vi "Process.vi"(0 "reference in":refnum<class "Grapher.lvclass">, 5 "error in":errorcluster) -> (14 "reference out":refnum<class "Grapher.lvclass">, 19 "error out":errorcluster)   [LabVIEW 2023, in "Grapher.lvclass"]
uses:
  Grapher.lvclass
  Grapher.lvclass/Grapher.ctl
  <vilib>/Utility/SystemLogging/NI_SystemLogging.lvlib
  <instrlib>/HPS-17000/HPS-17000.lvclass
  <vilib>/HPS-17000/MStream_grpc_CyclerMeasurement.ctl
  <vilib>/HPS-17000/NI_BC_client.lvlib
  Types/Indicators.ctl
panel:
  out "error info":errorcluster
  out "Last Command":string
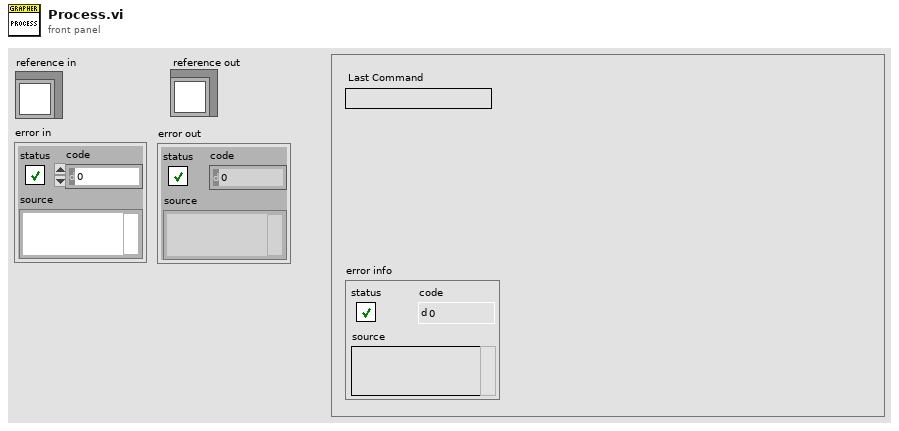
[diagram p1: front panel]
types:
  T1 = typedef "Indicators.ctl" = cluster{"XY Graph":refnum<vi>, "Voltage":refnum<vi>, "Current":refnum<vi>, "Power":refnum<vi>, "Function":refnum<vi>, "Charging":refnum<vi>, "Discharging":refnum<vi>}
  T2 = cluster{"Core":cluster{"Timeout":i32, "Events":cluster{"EventsToProcess":refnum<event-registration>}, "EventFromProcess":refnum<user-event>, "ProcessSyncQueue":refnum<queue>, "QueueFromProcess":refnum<queue>, "Command":string, "Data":variant}, "Chart History":cluster{"local timestamp":dbl[], "system timestamp":dbl[], "measured voltage":dbl[], "measured current":dbl[], "setpoint voltage":dbl[], "setpoint current":dbl[]}, "HPS17K Refs":refnum<class "HPS-17000.lvclass">[], "Use Local Time?":bool, "Graph Samples":u32, "Graph Decimation":i32, "High Speed?":bool, "Graph Queue":refnum<queue>, "Indicator Refs":T1, "Pause?":bool}
  T3 = cluster{"local timestamp":dbl[], "system timestamp":dbl[], "measured voltage":dbl[], "measured current":dbl[], "setpoint voltage":dbl[], "setpoint current":dbl[]}
  T4 = enum32{"Invalid", "Standard", "Closed", "Hidden", "Minimized", "Maximized"}
  T5 = cluster{"EventsToProcess":refnum<event-registration>}
  T6 = typedef "NI_BC_client.lvlib/MStream_grpc_CyclerMeasurement.ctl" = cluster{"measured_voltage":sgl, "measured_current":sgl, "setpoint_voltage":sgl, "setpoint_current":sgl, "timestamp":i64}
  T7 = typedef "Function.ctl" = enum16{"REGEN (LOAD)", "STANDBY", "SUPPLY (SOURCE)"}
  T8 = cluster{"system timestamp":dbl[], "measured voltage":dbl[]}
  T9 = cluster{"system timestamp":dbl[], "setpoint voltage":dbl[]}
  T10 = cluster{"system timestamp":dbl[], "measured current":dbl[]}
  T11 = cluster{"system timestamp":dbl[], "setpoint current":dbl[]}
  T12 = cluster{"system timestamp":dbl[], "setpoint current":dbl[]}[]
  T13 = typedef "Grapher.lvclass/ObjectAttributes.ctl" = cluster{"Indicator Refs":T1, "Update Rate (ms)":i32, "Graph Queue":refnum<queue>, "HPS17K Refs":refnum<class "HPS-17000.lvclass">[]}
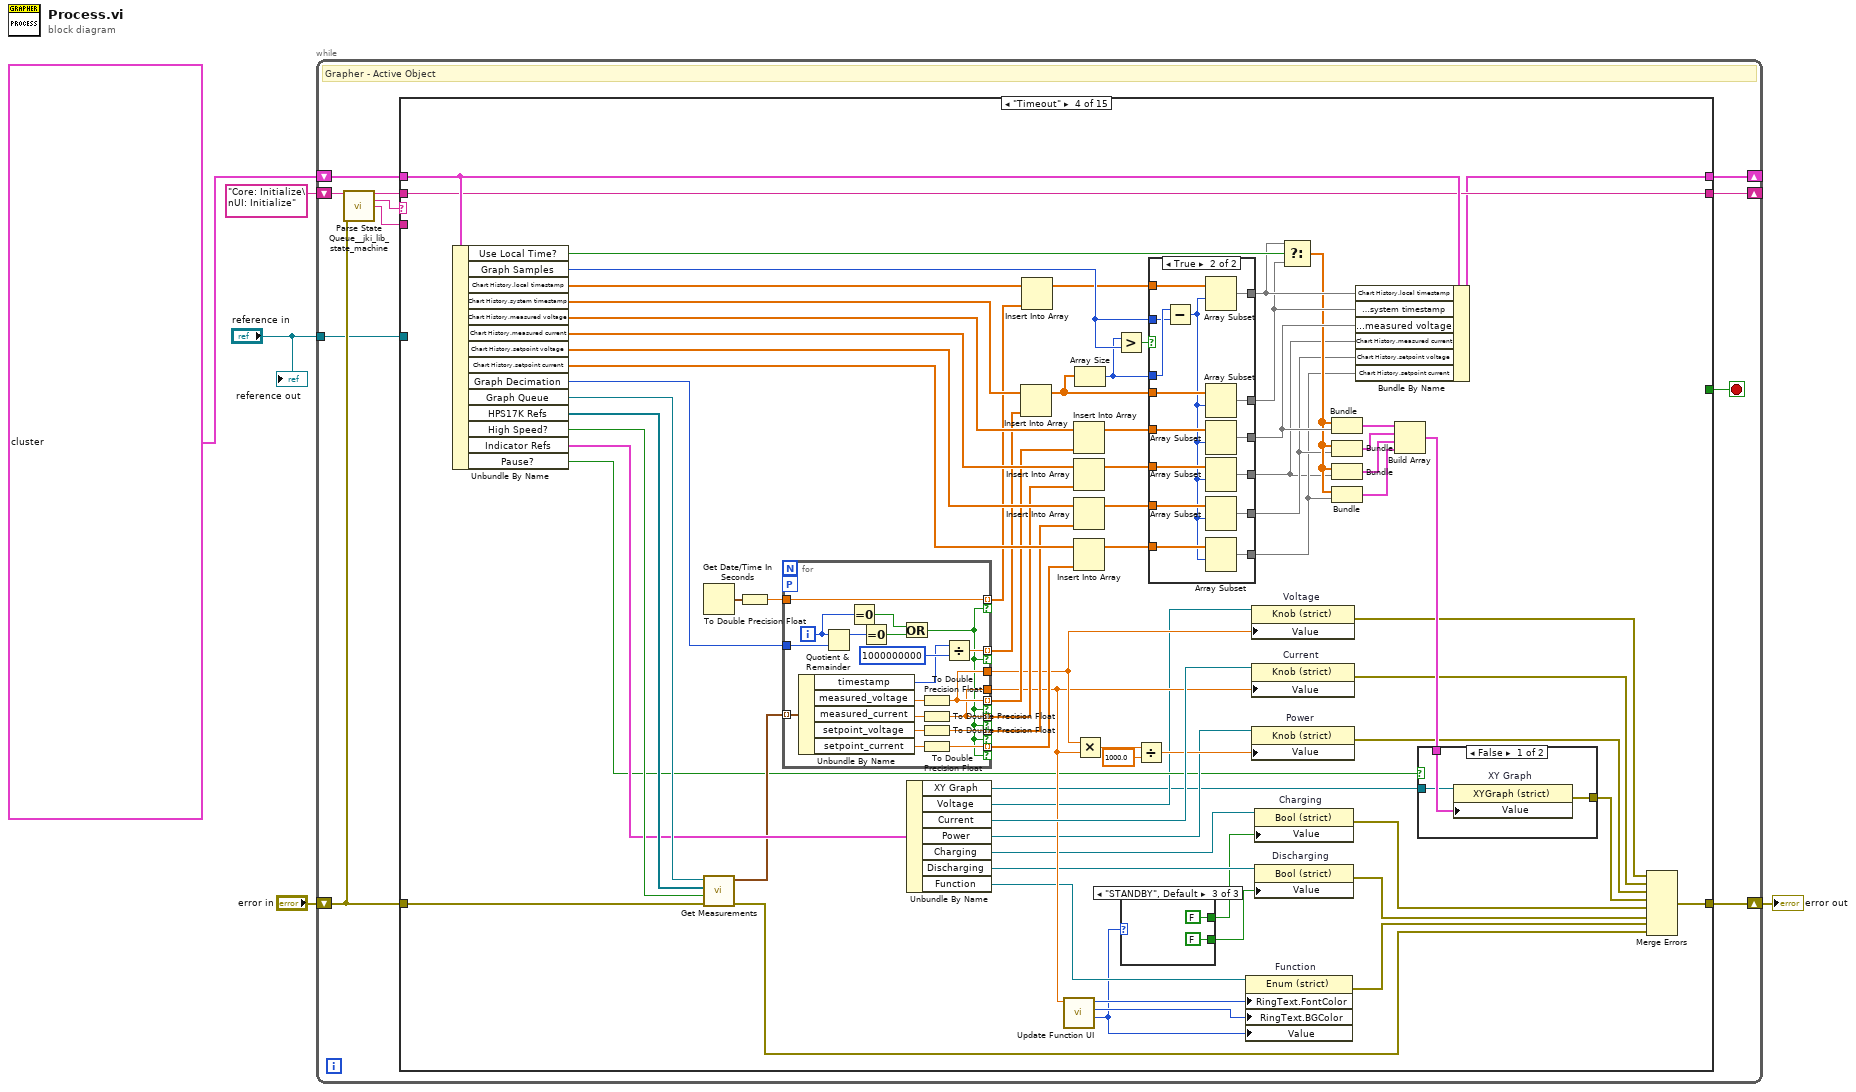
[diagram p0: block diagram]
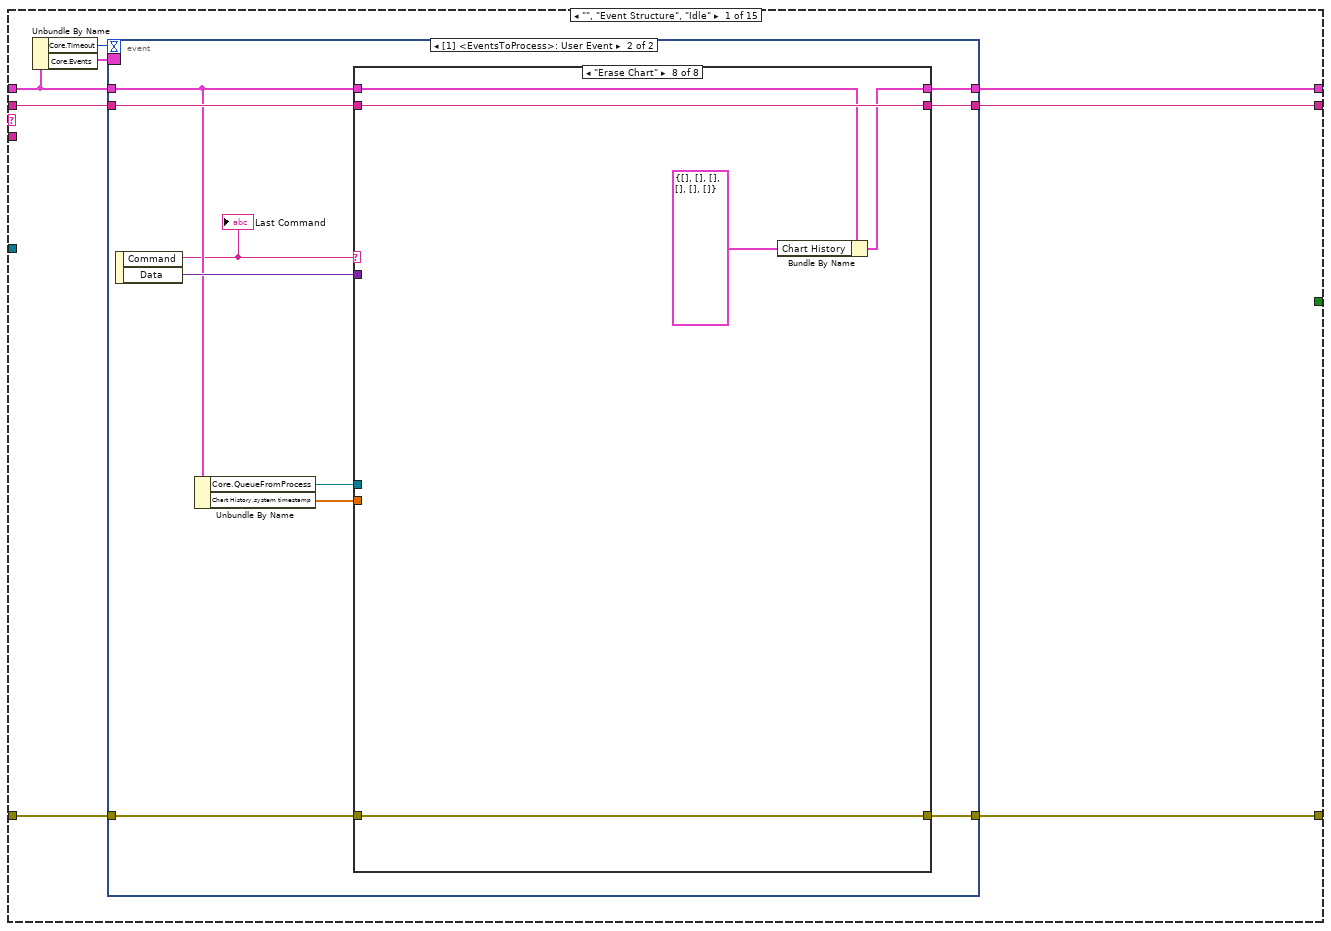
[diagram p2: hidden frame]
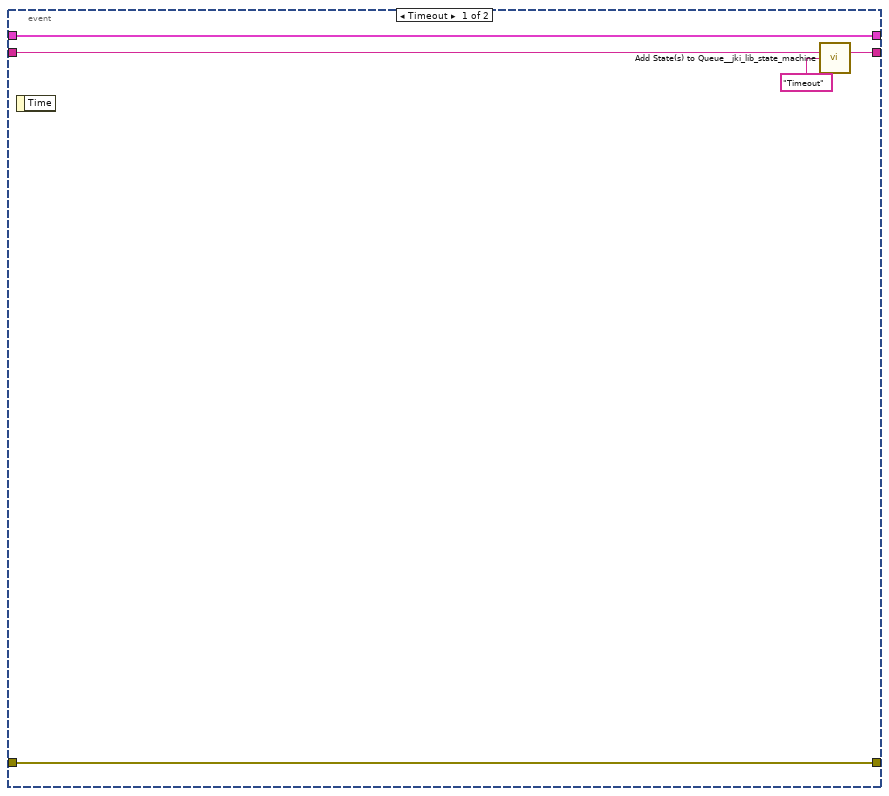
[diagram p3: hidden frame]
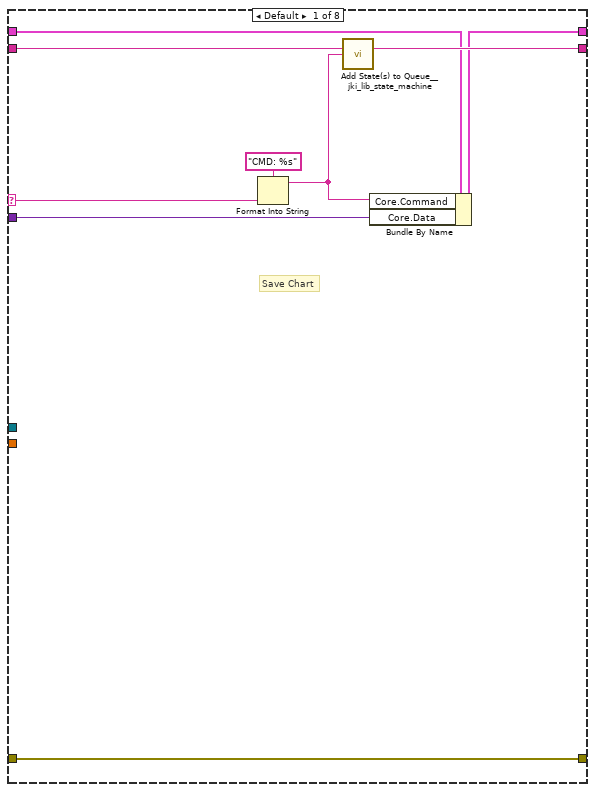
[diagram p4: hidden frame]
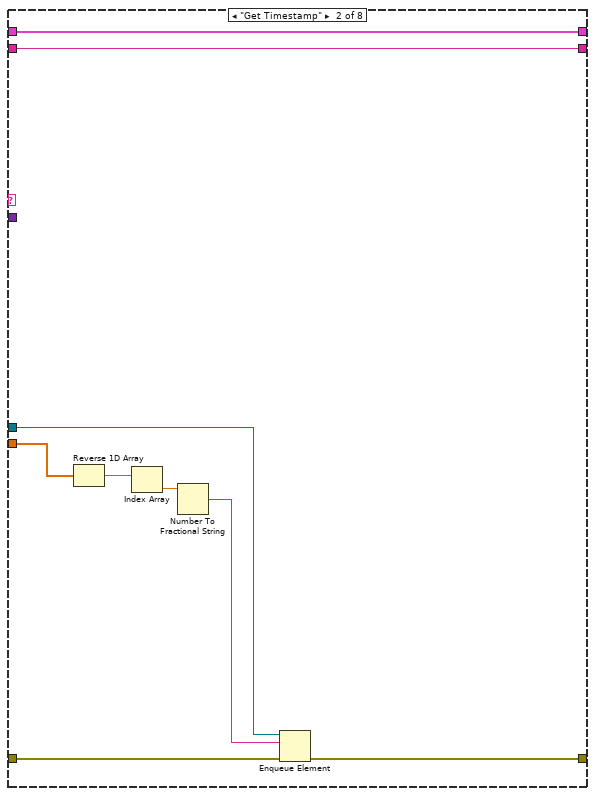
[diagram p5: hidden frame]
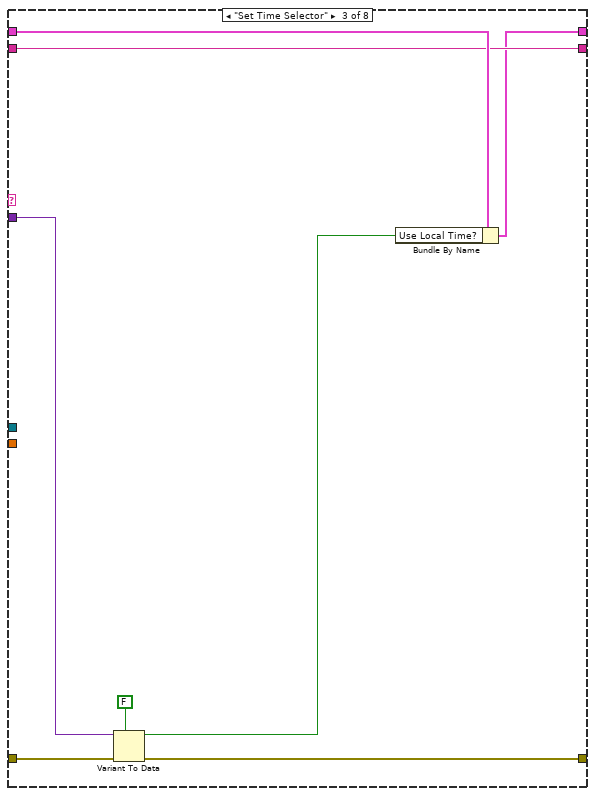
[diagram p6: hidden frame]
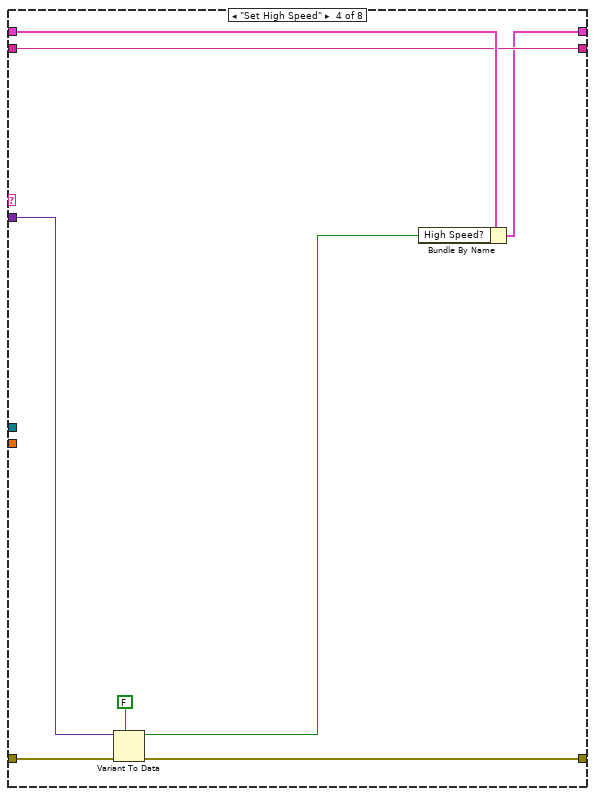
[diagram p7: hidden frame]
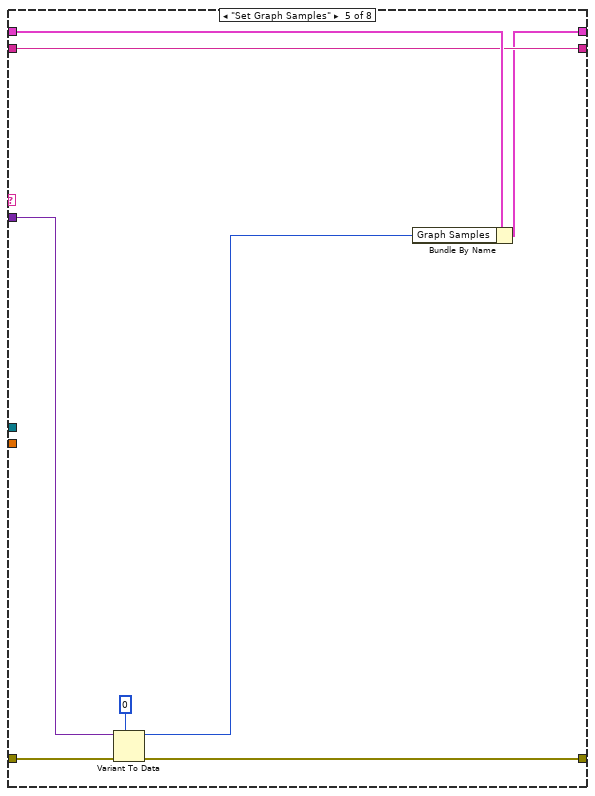
[diagram p8: hidden frame]
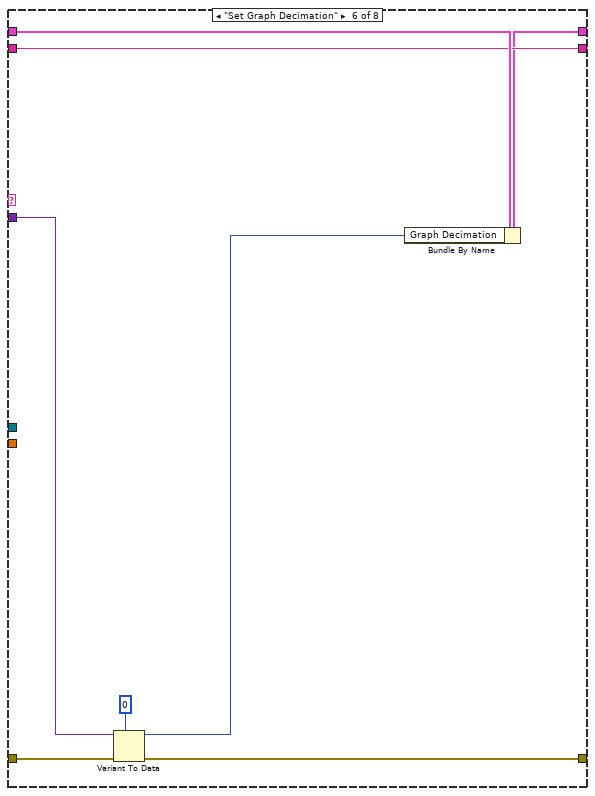
[diagram p9: hidden frame]
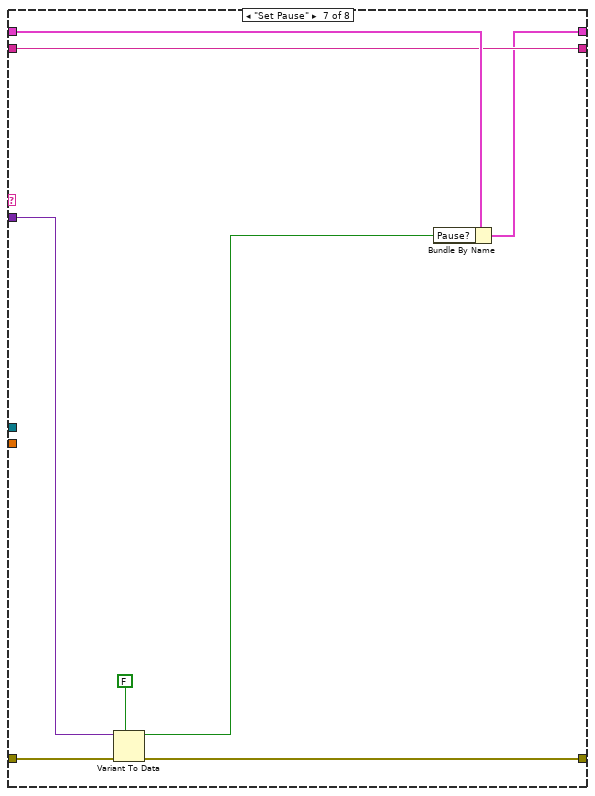
[diagram p10: hidden frame]
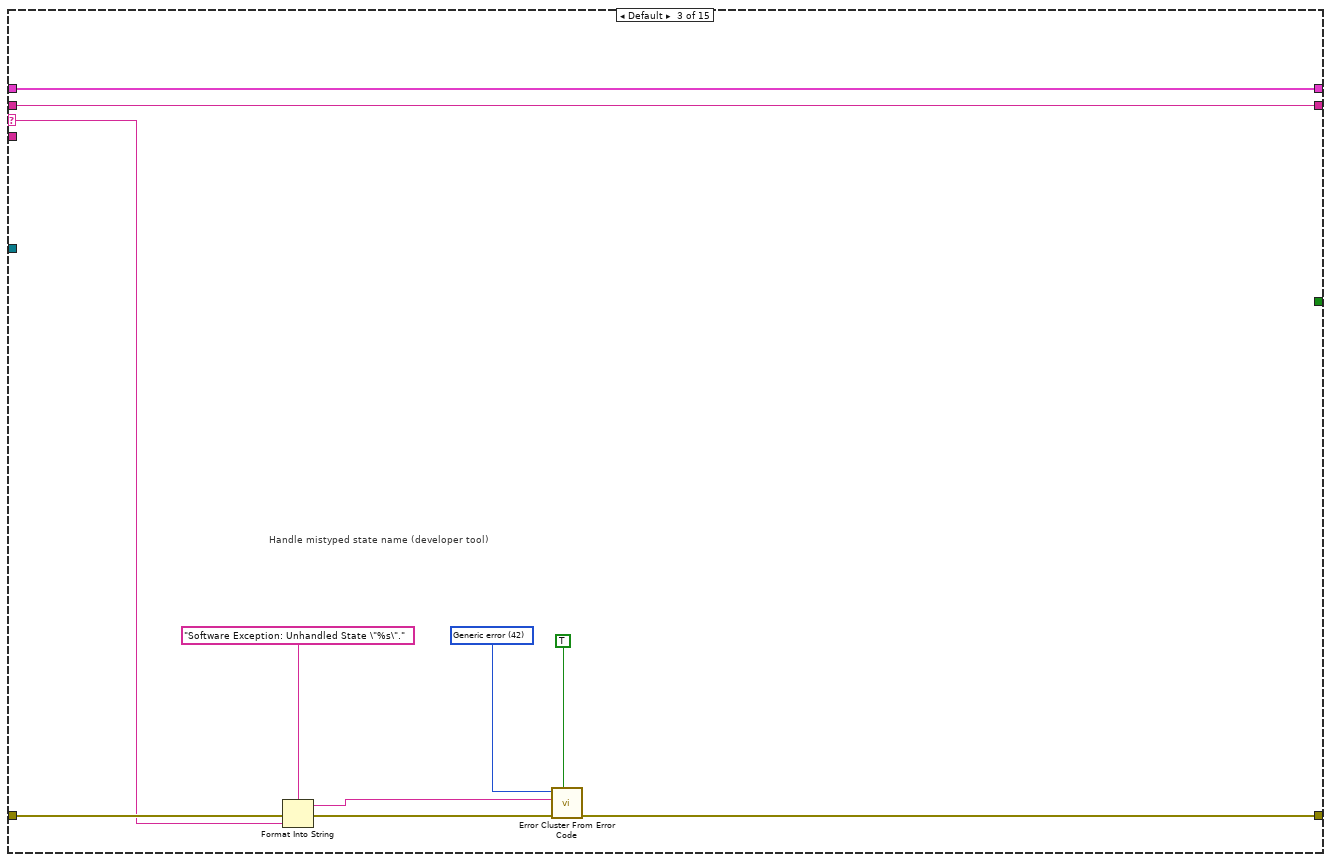
[diagram p12: hidden frame]
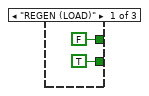
[diagram p13: hidden frame]
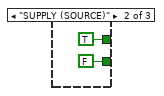
[diagram p14: hidden frame]
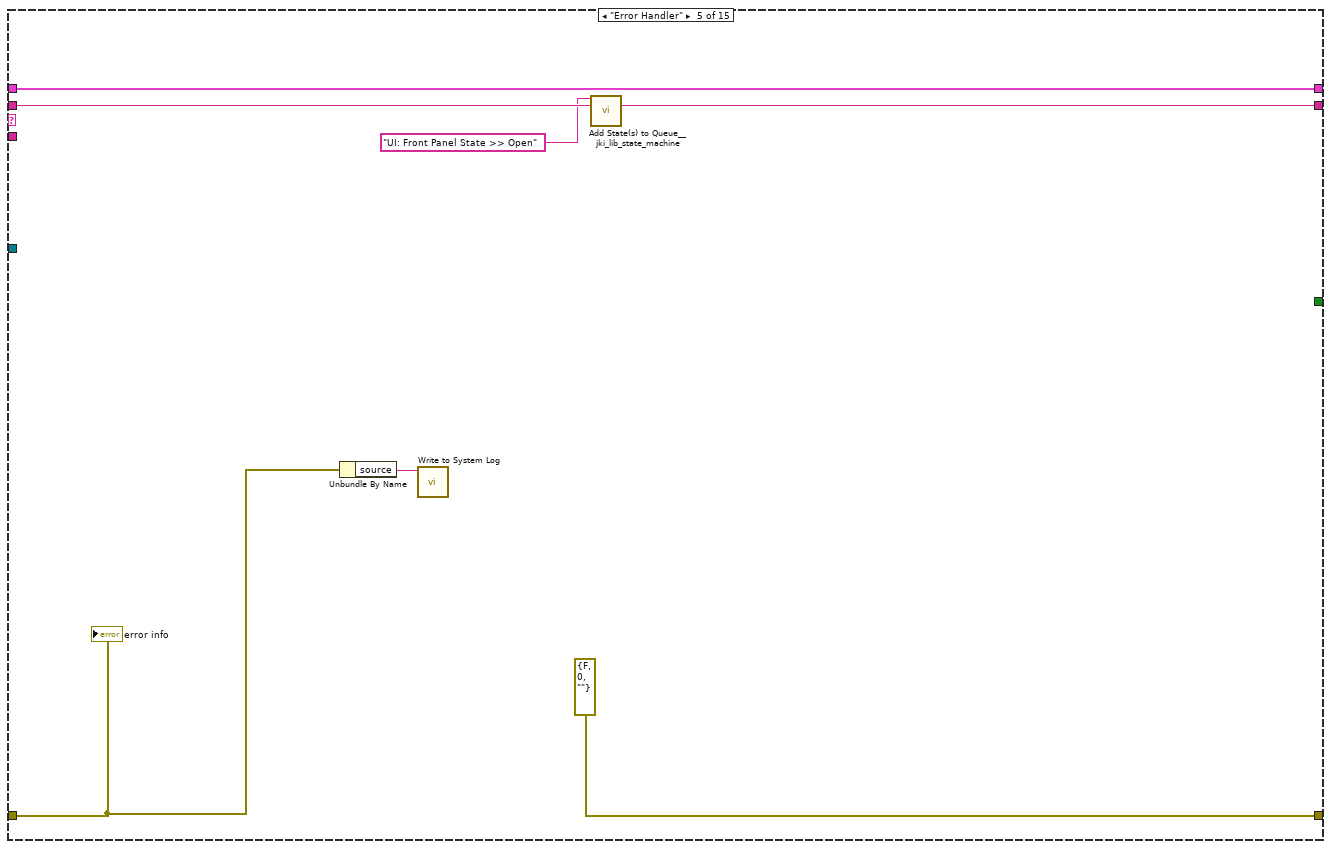
[diagram p17: hidden frame]
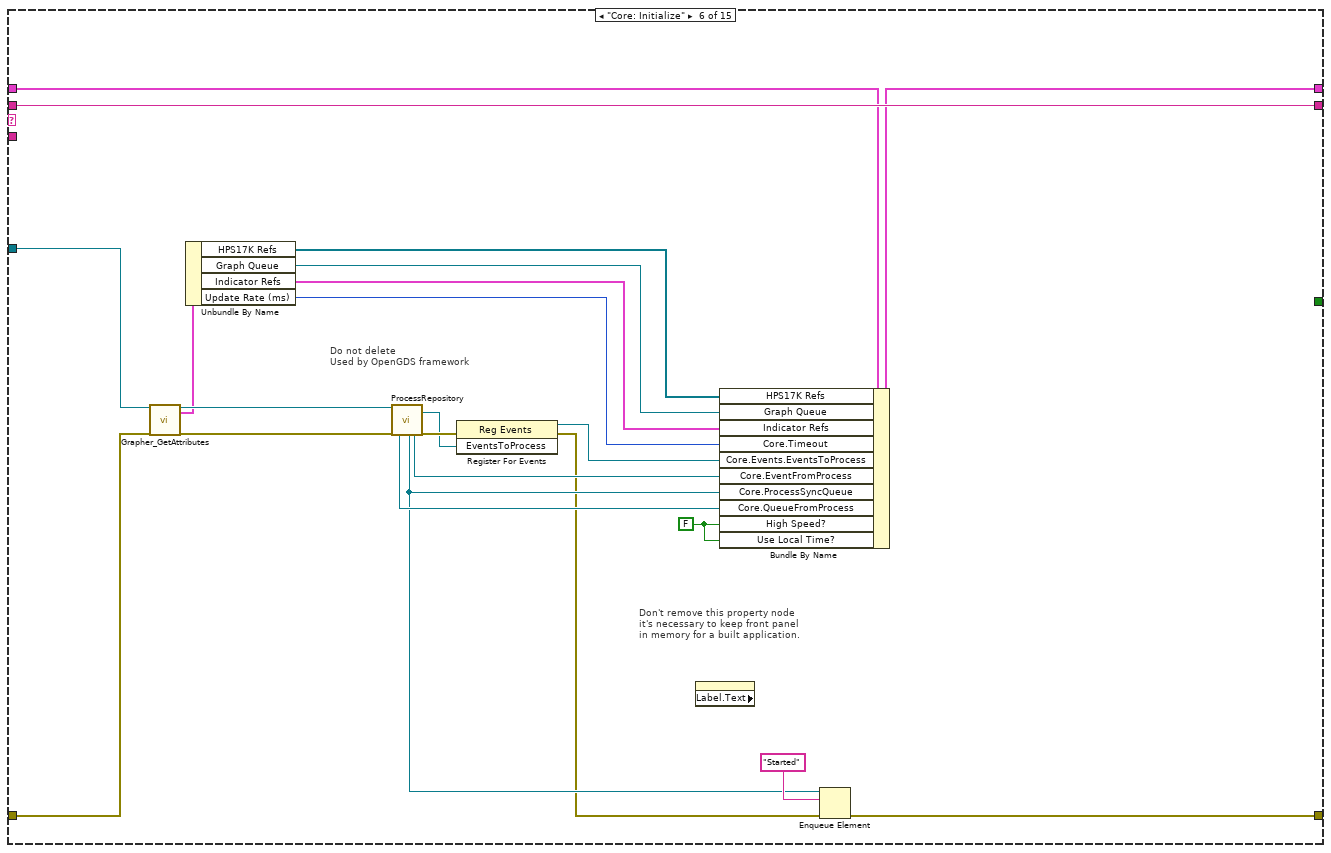
[diagram p18: hidden frame]
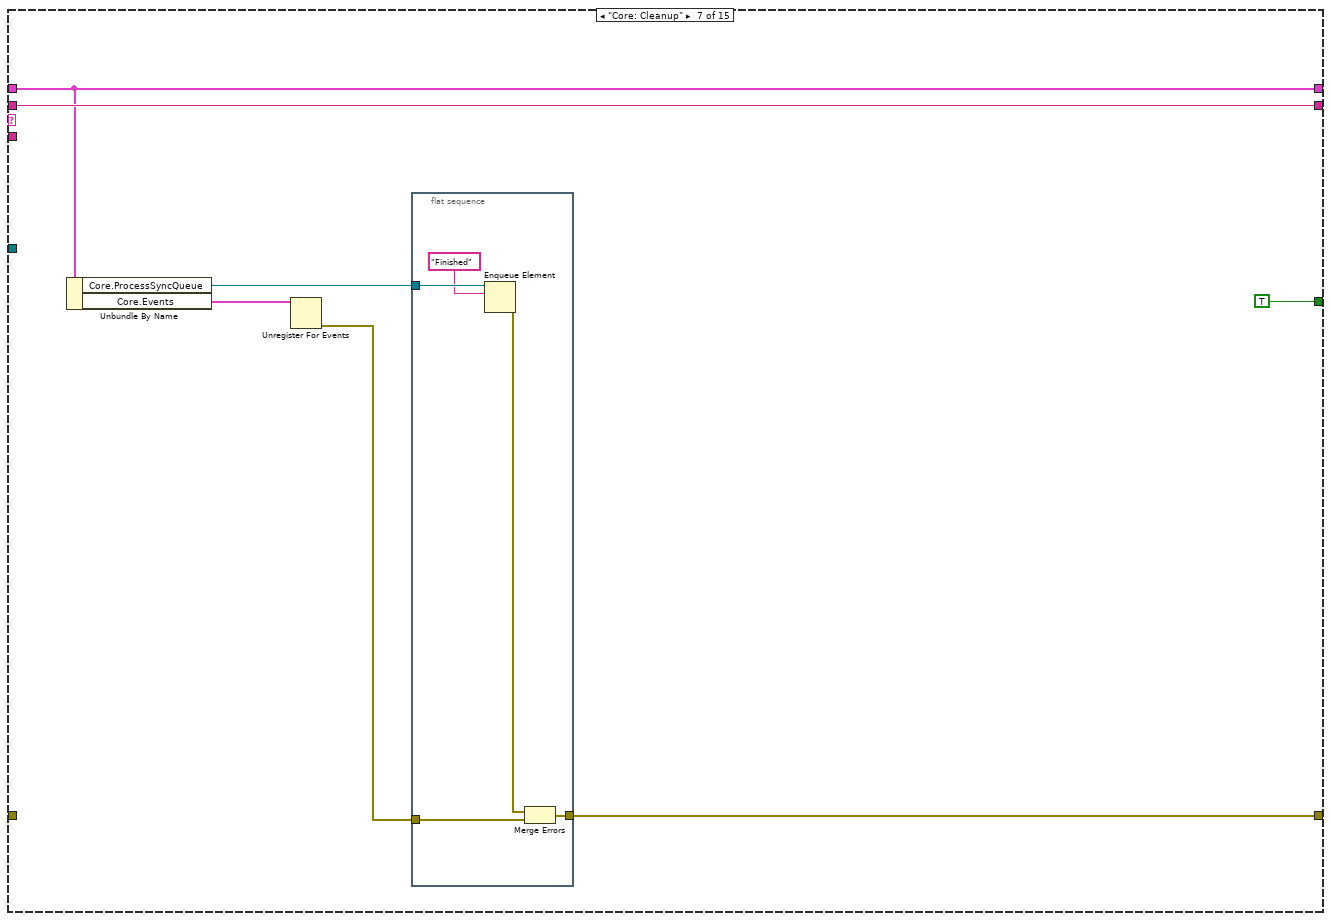
[diagram p19: hidden frame]
diagram:
  n1 = while {
    shift-right: [w15] -> w4
    shift-left: "error in" -> [w16]
    shift-right: [w8] -> _
    shift-left: "Core: Initialize\nUI: Initialize" ("States Out") -> [w11]
    shift-right: [w14] -> _
    shift-left: T2 {"Core"={"Timeout"=-1, "Events"={"EventsToProcess"=refnum}, "EventFromProcess"=refnum, "ProcessSyncQueue"=refnum, "QueueFromProcess"=refnum, "Command"="", "Data"=variant}, "Chart History"={"local timestamp"=[], "system timestamp"=[], "measured voltage"=[], "measured current"=[], "setpoint voltage"=[], "setpoint current"=[]}, "HPS17K Refs"=[], "Use Local Time?"=FALSE, "Graph Samples"=1000, "Graph Decimation"=1000, "High Speed?"=FALSE, "Graph Queue"=refnum, "Indicator Refs"={"XY Graph"=refnum, "Voltage"=refnum, "Current"=refnum, "Power"=refnum, "Function"=refnum, "Charging"=refnum, "Discharging"=refnum}, "Pause?"=FALSE} ("LocalVariables") -> [w13]
    tunnel: "reference in" -> [w6]
    stop <- w7 stop-if-true
    # "Grapher - Active Object"
    n2 = call <vilib>:"Parse State Queue__jki_lib_state_machine.vi"("State Queue"=w11, "Error In (no error)"=w16) -> ("Remaining States"=w10:string, "Current State"=w12:string, "Arguments"=w9:string)  [unwired: 11 in]
    n3 = case shown="\"Timeout\"" w12 {
      selector: w12 -> [_ _ w106 _ _ _ _ _ _ _ _ _ _ _ _]
      tunnel: w16 -> [w18 w105 w108 w187 w240 w254 _ w281 w282 w305 _ w312 w315 w322 w324]
      tunnel: [w19 w105 w107 w186 errorcluster {"status"=FALSE, "code"=0, "source"=""} ("error constant") w266 w269 w281 w282 w305 w306 w312 w315 w322 w323] -> w15
      tunnel: [w24 w104 w115 w184 w244 w264 w270 w280 w284 w297 w307 w311 w314 w321 w326] -> w14
      tunnel: w13 -> [w20 w104 w115 w188 w244 w263 w270 w280 w284 w297 w307 w311 w314 w321 w326]
      tunnel: w10 -> [w22 w103 w114 w185 w243 w265 w273 w279 w285 w304 w309 w310 _ w320 w327]
      tunnel: w9 -> [_ _ _ _ _ _ _ _ w283 _ _ _ _ w317 _]
      tunnel: [w21 w103 w114 w185 w242 w265 w273 w279 w285 w304 w309 w310 "UI: Cleanup\nCore: Cleanup" ("State(s) at Back (\"\")") w319 w327] -> w8
      tunnel: [_ _ _ _ _ _ TRUE _ _ _ _ _ _ _ _] -> w7
      tunnel: w6 -> [_ _ _ _ _ w252 _ _ _ _ _ _ _ _ _]
      frame "", "Event Structure", "Idle" {
        n4 = Unbundle By Name(w20) -> ("Core.Timeout"=w17:i32, "Core.Events"=w23:T5)
        n5 = event shown="[1] <EventsToProcess>: User Event" {
          selector: w23 -> [_ _]
          dyn-events: _ -> [_ _]
          timeout: w17 -> [_ _]
          tunnel: w20 -> [w29 w34]
          tunnel: [w29 w37] -> w24
          tunnel: [w27 w39] -> w21
          tunnel: w22 -> [w28 w38]
          tunnel: [w25 w30] -> w19
          tunnel: w18 -> [w25 w31]
          event Timeout {
            n6 = event-data() -> ()  [unwired: 1 in, 1 out]
            n7 = call <vilib>:"Add State(s) to Queue__jki_lib_state_machine.vi"("State(s) in (\"\")"=w28, "State(s) at Back (\"\")"="Timeout" ("State(s) at Back (\"\")")) -> ("States Out"=w27:string)  [unwired: 13 in]
          }
          event User Event {
            n8 = event-data() -> ("Command"=w33:string, "Data"=w36:variant)  [unwired: 1 in]
            "Last Command" <- w33
            n9 = Unbundle By Name(w34) -> ("Core.QueueFromProcess"=w35:refnum<queue>, "Chart History.system timestamp"=w32:dbl[])
            n10 = case shown="\"Erase Chart\"" w33 {
              selector: w33 -> [w41 _ _ _ _ _ _ _]
              tunnel: [w48 w55 w62 w70 w78 w86 w94 w102] -> w39
              tunnel: w38 -> [w47 w55 w62 w70 w78 w86 w94 w102]
              tunnel: [w46 w56 w59 w67 w77 w85 w93 w100] -> w37
              tunnel: w36 -> [w45 _ w64 w72 w80 w88 w96 _]
              tunnel: w35 -> [_ w57 _ _ _ _ _ _]
              tunnel: w34 -> [w44 w56 w63 w71 w79 w87 w95 w101]
              tunnel: w32 -> [_ w53 _ _ _ _ _ _]
              tunnel: w31 -> [w40 w54 w65 w73 w81 w89 w97 w99]
              tunnel: [w40 w49 w58 w66 w76 w84 w92 w99] -> w30
              frame Default {
                # "Save Chart"
                n11 = Format Into String(format string="CMD: %s", w41) -> (resulting string=w42:string)  [unwired: 2 in, 1 out]
                n12 = call <vilib>:"Add State(s) to Queue__jki_lib_state_machine.vi"("State(s) in (\"\")"=w47, "State(s) at Back (\"\")"=w42) -> ("States Out"=w48:string)  [unwired: 13 in]
                n13 = Bundle By Name(cluster=w44, "Core.Command"=w42, "Core.Data"=w45) -> (w46:T2)
              }
              frame "Get Timestamp" {
                n14 = Reverse 1D Array(array=w53) -> (reversed array=w52:dbl[])
                n15 = Index Array(array=w52) -> (element=w51:dbl)  [unwired: 1 in]
                n16 = Number To Fractional String(number=w51) -> (F-format string=w50:string)  [unwired: 3 in]
                n17 = Enqueue Element ("Return message to the client from this process")(queue=w57, element=w50, error in (no error)=w54) -> (error out=w49:errorcluster)  [unwired: 1 in, 2 out]
              }
              frame "Set Time Selector" {
                n18 = Variant To Data(error in=w65, type=FALSE, Variant=w64) -> (data=w61:bool, error out=w58:errorcluster)
                n19 = Bundle By Name(cluster=w63, "Use Local Time?"=w61) -> (w59:T2)
              }
              frame "Set High Speed" {
                n20 = Variant To Data(error in=w73, type=FALSE, Variant=w72) -> (data=w69:bool, error out=w66:errorcluster)
                n21 = Bundle By Name(cluster=w71, "High Speed?"=w69) -> (w67:T2)
              }
              frame "Set Graph Samples" {
                n22 = Variant To Data(error in=w81, type=u32 0 ("Graph Samples"), Variant=w80) -> (data=w74:u32, error out=w76:errorcluster)
                n23 = Bundle By Name(cluster=w79, "Graph Samples"=w74) -> (w77:T2)
              }
              frame "Set Graph Decimation" {
                n24 = Variant To Data(error in=w89, type=0 ("Graph Samples"), Variant=w88) -> (data=w82:i32, error out=w84:errorcluster)
                n25 = Bundle By Name(cluster=w87, "Graph Decimation"=w82) -> (w85:T2)
              }
              frame "Set Pause" {
                n26 = Variant To Data(error in=w97, type=FALSE, Variant=w96) -> (data=w91:bool, error out=w92:errorcluster)
                n27 = Bundle By Name(cluster=w95, "Pause?"=w91) -> (w93:T2)
              }
              frame "Erase Chart" {
                n28 = Bundle By Name(cluster=w101, "Chart History"=T3 {"local timestamp"=[], "system timestamp"=[], "measured voltage"=[], "measured current"=[], "setpoint voltage"=[], "setpoint current"=[]}) -> (w100:T2)
              }
            }
          }
        }
      }
      frame "---------- Core ----------" {
      }
      frame Default {
        w112 = 42 items=["No error", "Argument error", "Memory is full", "Out of zone", "End of file", "File already open", "Generic file I/O error", "File not found", "File permission error", "Disk is full", "Duplicate path", "Too many files open", "System feature not enabled", "Resource file not found", "Cannot add resource", "Resource not found", "Image not found", "Image memory error", "Pen does not exist", "Config type invalid", "Config token not found", "Config parse error", "Config memory error", "Bad external code format", "Bad external code offset", "External code not present", "Null window", "Destroy window error", "Null menu", "Print aborted", "Bad print record", "Print driver error", "Windows error during printing", "Memory error during printing", "Print dialog error", "Generic print error", "Invalid device refnum", "Device not found", "Device parameter error", "Device unit error", "Cannot open device", "Device call aborted", "Generic error", "Cancelled by user", "Object ID too low", "Object ID too high", "Object not in heap", "Unknown heap", "Unknown object (invalid DefProc)", "Unknown object (DefProc not in table)", "Message out of range", "Invalid (null) method", "Unknown message", "Manager call not supported", "Bad address", "Network operation in progress", "Network operation timed out", "Connection is busy", "Network attribute not supported", "Network error", "Address in use", "System out of memory", "Connection aborted", "Connection refused", "Not connected", "Already connected", "Connection closed", "Initialization error (interapplication manager)", "Bad occurrence", "Wait on unbound occurrence handler", "Occurrence queue overflow", "Datalog type conflict", "Unused", "Unrecognized type (interapplication manager)", "Memory corrupt", "Failed to make temporary DLL", "Old CIN version", "Drag socket not found", "Failed to load drop-object", "Failed to register OLE object", "Failed to release OLE object", "Format specifier type mismatch", "Unknown format specifier", "Too few format specifiers", "Too many format specifiers", "Scan failed", "Newer CIN version", "Error converting to variant", "Runtime menu error", "Password tampered", "Variant attribute not found", "Incompatible variant data type", "Event data is not available", "Event Store is not present", "Occurrence is not found", "Event Queue is not created", "Event info is not available", "Refnum passed is NULL", "Error retrieving Class GUID", "Error retrieving CoClass GUID", "Error retrieving TypeLib GUID.", "Bad built application magic bytes.", "Specific driver is different from the specific driver associated with the Logical Name.", "There is no session opened to the class driver.", "Max Error", "MAX - Error with config objects", "MAX - Error loading configuration", "MAX - Group not supported"]
        # "Handle mistyped state name (developer tool)"
        n29 = Format Into String(format string="Software Exception: Unhandled State \"%s\"." ("message"), error in=w108, w106) -> (resulting string=w111:string, error out=w110:errorcluster)  [unwired: 1 in]
        n30 = call <vilib>:"Error Cluster From Error Code.vi"("show call chain? (False)"=TRUE, "error in (no error)"=w110, "error message (\"\")"=w111, "error code (0)"=w112) -> ("error out"=w107:errorcluster)  [unwired: 5 in]
      }
      frame "Timeout" {
        n31 = Unbundle By Name(w188) -> ("Use Local Time?"=w171:bool, "Graph Samples"=w183:u32, "Chart History.local timestamp"=w182:dbl[], "Chart History.system timestamp"=w181:dbl[], "Chart History.measured voltage"=w180:dbl[], "Chart History.measured current"=w179:dbl[], "Chart History.setpoint voltage"=w178:dbl[], "Chart History.setpoint current"=w177:dbl[], "Graph Decimation"=w176:i32, "Graph Queue"=w175:refnum<queue>, "HPS17K Refs"=w174:refnum<class "HPS-17000.lvclass">[], "High Speed?"=w173:bool, "Indicator Refs"=w172:T1, "Pause?"=w128:bool)
        n32 = Get Date/Time In Seconds() -> (seconds since 1Jan1904=w163:timestamp)
        n33 = call "Get Measurements.vi"("error in (no error)"=w187, "High Speed"=w173, "HPS17K Refs"=w174, "Stream Queue"=w175) -> ("error out"=w122:errorcluster, "Measurements"=w148:T6[])  [unwired: 6 in]
        n34 = To Double Precision Float(number=w163) -> (double precision float=w142:dbl)
        n35 = for {
          tunnel: w148 -> [w216] mode=indexing
          tunnel: [w206] -> w143 mode=indexing if=w198
          tunnel: [w205] -> w144 mode=indexing if=w198
          tunnel: [w210] -> w154 mode=indexing if=w198
          tunnel: [w209] -> w153 mode=indexing if=w198
          tunnel: [w207] -> w149 mode=indexing if=w198
          workers-P: _ -> [_]
          tunnel: [w206] -> w137
          tunnel: [w205] -> w135
          tunnel: w176 -> [w204]
          tunnel: w142 -> [w199]
          tunnel: [w199] -> w141 mode=indexing if=w198
          i -> [w201]
          n36 = Unbundle By Name(w216) -> ("timestamp"=w208:i64, "measured_voltage"=w214:sgl, "measured_current"=w213:sgl, "setpoint_voltage"=w212:sgl, "setpoint_current"=w211:sgl)
          n37 = Quotient & Remainder(x=w201, y=w204) -> (x-y*floor(x/y)=w203:i32)  [unwired: 1 out]
          n38 = Equal To 0?(x=w201) -> (x = 0?=w200:bool)
          n39 = Equal To 0?(x=w203) -> (x = 0?=w202:bool)
          n40 = Or(x=w200, y=w202) -> (x .or. y?=w198:bool)
          n41 = To Double Precision Float(number=w214) -> (double precision float=w206:dbl)
          n42 = To Double Precision Float(number=w213) -> (double precision float=w205:dbl)
          n43 = To Double Precision Float(number=w212) -> (double precision float=w207:dbl)
          n44 = To Double Precision Float(number=w211) -> (double precision float=w210:dbl)
          n45 = Divide(x=w208, y=i64 1000000000) -> (x/y=w209:dbl)
        }
        n46 = Unbundle By Name(w172) -> ("XY Graph"=w124:refnum<vi>, "Voltage"=w125:refnum<vi>, "Current"=w136:refnum<vi>, "Power"=w133:refnum<vi>, "Charging"=w123:refnum<vi>, "Discharging"=w126:refnum<vi>, "Function"=w127:refnum<vi>)
        n47 = Insert Into Array(array=w181, new element=w153) -> (w151:dbl[])  [unwired: 1 in]
        n48 = Insert Into Array(array=w182, new element=w141) -> (w152:dbl[])  [unwired: 1 in]
        n49 = call "Update Function UI.vi"("measured_current"=w135) -> ("Function"=w118:T7, "BG Color"=w139:u32, "Font Color"=w140:u32)  [unwired: 8 in]
        n50 = Insert Into Array(array=w180, new element=w143) -> (w158:dbl[])  [unwired: 1 in]
        n51 = Insert Into Array(array=w179, new element=w144) -> (w157:dbl[])  [unwired: 1 in]
        n52 = Insert Into Array(array=w178, new element=w149) -> (w156:dbl[])  [unwired: 1 in]
        n53 = Insert Into Array(array=w177, new element=w154) -> (w155:dbl[])  [unwired: 1 in]
        n54 = Array Size(array=w151) -> (size(s)=w150:i32)
        n55 = Multiply(x=w137, y=w135) -> (x*y=w170:dbl)
        n56 = Greater?(x=w150, y=w183) -> (0:w159:bool)
        n57 = case shown="\"STANDBY\", Default" w118 {
          tunnel: [TRUE FALSE FALSE] -> w117
          tunnel: [FALSE TRUE FALSE] -> w116
          frame "REGEN (LOAD)" {
          }
          frame "SUPPLY (SOURCE)" {
          }
          frame "STANDBY", Default {
          }
        }
        n58 = Divide(x=w170, y=1000.0) -> (x/y=w134:dbl)
        n59 = case shown="True" w159 {
          tunnel: w151 -> [w222 w233]
          tunnel: w158 -> [w221 w231]
          tunnel: w157 -> [w220 w229]
          tunnel: w156 -> [w219 w227]
          tunnel: w155 -> [w218 w226]
          tunnel: [w218 w225] -> w146
          tunnel: [w219 w224] -> w147
          tunnel: [w220 w228] -> w145
          tunnel: [w221 w230] -> w164
          tunnel: [w222 w232] -> w161
          tunnel: w152 -> [w217 w235]
          tunnel: [w217 w234] -> w162
          tunnel: w150 -> [_ w237]
          tunnel: w183 -> [_ w236]
          frame False {
          }
          frame True {
            n60 = Subtract(x=w237, y=w236) -> (x-y=w223:u32)
            n61 = Array Subset(array=w235, index=w223) -> (w234:dbl[])  [unwired: 1 in]
            n62 = Array Subset(array=w233, index=w223) -> (w232:dbl[])  [unwired: 1 in]
            n63 = Array Subset(array=w231, index=w223) -> (w230:dbl[])  [unwired: 1 in]
            n64 = Array Subset(array=w229, index=w223) -> (w228:dbl[])  [unwired: 1 in]
            n65 = Array Subset(array=w227, index=w223) -> (w224:dbl[])  [unwired: 1 in]
            n66 = Array Subset(array=w226, index=w223) -> (w225:dbl[])  [unwired: 1 in]
          }
        }
        n67 = property on="Function" class="Enum (strict)"(reference=w127, "RingText.FontColor"=w140, "RingText.BGColor"=w139, "Value"=w118) -> (error out=w121:errorcluster)  [unwired: 1 in, 1 out]
        n68 = property on="Voltage" class="Knob (strict)"(reference=w125, "Value"=w137) -> (error out=w129:errorcluster)  [unwired: 1 in, 1 out]
        n69 = property on="Current" class="Knob (strict)"(reference=w136, "Value"=w135) -> (error out=w130:errorcluster)  [unwired: 1 in, 1 out]
        n70 = property on="Power" class="Knob (strict)"(reference=w133, "Value"=w134) -> (error out=w131:errorcluster)  [unwired: 1 in, 1 out]
        n71 = property on="Charging" class="Bool (strict)"(reference=w123, "Value"=w116) -> (error out=w119:errorcluster)  [unwired: 1 in, 1 out]
        n72 = property on="Discharging" class="Bool (strict)"(reference=w126, "Value"=w117) -> (error out=w120:errorcluster)  [unwired: 1 in, 1 out]
        n73 = Select(t=w162, s=w171, f=w161) -> (s? t:f=w160:dbl[])
        n74 = Bundle("system timestamp"=w160, "measured voltage"=w164) -> (w168:T8)  [unwired: 1 in]
        n75 = Bundle("system timestamp"=w160, "setpoint voltage"=w147) -> (w167:T9)  [unwired: 1 in]
        n76 = Bundle("system timestamp"=w160, "measured current"=w145) -> (w166:T10)  [unwired: 1 in]
        n77 = Bundle("system timestamp"=w160, "setpoint current"=w146) -> (w165:T11)  [unwired: 1 in]
        n78 = Bundle By Name(cluster=w188, "Chart History.local timestamp"=w162, "Chart History.system timestamp"=w161, "Chart History.measured voltage"=w164, "Chart History.measured current"=w145, "Chart History.setpoint voltage"=w147, "Chart History.setpoint current"=w146) -> (w184:T2)
        n79 = Build Array(w168, w167, w166, w165) -> (w138:T12)
        n80 = case shown="False" w128 {
          tunnel: w138 -> [w197 _]
          tunnel: w124 -> [w196 _]
          tunnel: [w195 _] -> w132
          frame False {
            n81 = property on="XY Graph" class="XYGraph (strict)"(reference=w196, "Value"=w197) -> (error out=w195:errorcluster)  [unwired: 1 in, 1 out]
          }
          frame True {
          }
        }
        n82 = Merge Errors(w129, w130, w131, w132, w119, w120, w121, w122) -> (w186:errorcluster)
      }
      frame "Error Handler" {
        n83 = Unbundle By Name(w240) -> ("source"=w238:string)
        n84 = call <vilib>:"Write to System Log.vi"("message"=w238) -> ()  [unwired: 10 in, 1 out]
        n85 = call <vilib>:"Add State(s) to Queue__jki_lib_state_machine.vi"("State(s) in Front (\"\")"="UI: Front Panel State >> Open" ("State(s) at Back (\"\")"), "State(s) in (\"\")"=w243) -> ("States Out"=w242:string)  [unwired: 13 in]
        "error info" <- w240
      }
      frame "Core: Initialize" {
        w245 = FALSE ("Connected?")
        # "Do not delete\nUsed by OpenGDS framework"
        # "Don't remove this property node\nit's necessary to keep front panel\nin memory for a built application."
        # "Template created by VI Technologies"
        n86 = call "Grapher_GetAttributes.vi"("reference in"=w252, "Error In"=w254) -> ("reference out"=w251:refnum<class "Grapher.lvclass">, "Data"=w250:T13, "Error Out"=w253:errorcluster)  [unwired: 14 in, 1 out]
        n87 = Unbundle By Name(w250) -> ("HPS17K Refs"=w246:refnum<class "HPS-17000.lvclass">[], "Graph Queue"=w247:refnum<queue>, "Indicator Refs"=w248:T1, "Update Rate (ms)"=w249:i32)
        n88 = call "ProcessRepository.vi"("reference in"=w251, "Error In"=w253) -> ("QueueFromProcess"=w258:refnum<queue>, "ProcessSyncQueue"=w256:refnum<queue>, "EventFromProcess"=w259:refnum<user-event>, "EventsToProcess"=w261:refnum<user-event>, "Error Out"=w262:errorcluster)  [unwired: 10 in, 3 out]
        n89 = register-events(error in=w262, w261) -> (reference out=w260:refnum<event-registration>, error out=w255:errorcluster)  [unwired: 1 in]
        n90 = property on="reference in" class="LVClassControl (strict)" props=["Label", "Text"]() -> ()  [unwired: 2 in, 3 out]
        n91 = Bundle By Name(cluster=w263, "HPS17K Refs"=w246, "Graph Queue"=w247, "Indicator Refs"=w248, "Core.Timeout"=w249, "Core.Events.EventsToProcess"=w260, "Core.EventFromProcess"=w259, "Core.ProcessSyncQueue"=w256, "Core.QueueFromProcess"=w258, "High Speed?"=w245, "Use Local Time?"=w245) -> (w264:T2)
        n92 = Enqueue Element(queue=w256, element="Started", error in (no error)=w255) -> (error out=w266:errorcluster)  [unwired: 1 in, 2 out]
      }
      frame "Core: Cleanup" {
        n93 = Unbundle By Name(w270) -> ("Core.ProcessSyncQueue"=w271:refnum<queue>, "Core.Events"=w268:T5)
        n94 = Unregister For Events(event registration refnum=w268) -> (error out=w267:errorcluster)  [unwired: 1 in]
        n95 = flat-sequence {
          tunnel: [w277] -> w269
          tunnel: w271 -> [w276]
          tunnel: w267 -> [w275]
          frame #0 {
            n96 = Enqueue Element(queue=w276, element="Finished") -> (error out=w278:errorcluster)  [unwired: 2 in, 2 out]
            n97 = Merge Errors(w278, w275) -> (w277:errorcluster)
          }
        }
      }
      frame "---------- UI ----------" {
      }
      frame "UI: Front Panel State" {
        n98 = case shown="\"Close\"" w283 {
          frame "Open", Default {
            n99 = property class="VI"() -> ("FP.State"=w286:T4)  [unwired: 2 in, 2 out]
            n100 = case shown="Default" w286 {
              frame Default {
                n101 = invoke class="VI" method="FP.Open"("Activate"=TRUE, "State"=T4."Standard") -> ()  [unwired: 3 in, 5 out]
              }
              frame "Standard" {
              }
            }
          }
          frame "Close" {
            n102 = property class="VI"() -> ("FP.State"=w289:T4)  [unwired: 2 in, 2 out]
            n103 = case shown="Default" w289 {
              frame "Closed" {
              }
              frame Default {
                n104 = invoke class="VI" method="FP.Close"() -> ()  [unwired: 3 in, 3 out]
              }
            }
          }
        }
      }
      frame "UI: Initialize" {
        n105 = property class="VI"() -> ("Name"=w303:string)  [unwired: 2 in, 2 out]
        n106 = Match Pattern(string=w303, regular expression="\\2Evi$") -> (before substring=w301:string)  [unwired: 1 in, 3 out]
        n107 = Reverse String(1:w301) -> (0:w300:string)
        n108 = Match Pattern(string=w300, regular expression=":") -> (before substring=w298:string, after substring=w296:string)  [unwired: 1 in, 2 out]
        n109 = Match Pattern(string=w296, regular expression="\\2E") -> (after substring=w294:string)  [unwired: 1 in, 3 out]
        n110 = Reverse String(1:w294) -> (0:w293:string)
        n111 = Reverse String(1:w298) -> (0:w292:string)
        n112 = Format Into String(format string="%s %s", w293, w292) -> (resulting string=w291:string)  [unwired: 2 in, 1 out]
        n113 = property class="VI"("Front Panel.Title"=w291) -> ()  [unwired: 2 in, 2 out]
      }
      frame "UI: Cleanup" {
        n114 = property class="VI"() -> (error out=w306:errorcluster, "FP.State"=w308:T4)  [unwired: 2 in, 1 out]
        n115 = case shown="\"Standard\", Default" w308 {
          frame "Closed" {
          }
          frame "Standard", Default {
            n116 = invoke class="VI" method="FP.Close"() -> ()  [unwired: 3 in, 3 out]
          }
        }
      }
      frame "---------- CMD ----------" {
      }
      frame "CMD: Exit" {
      }
      frame "CMD: Front Panel State" {
        n117 = Format Into String(format string="UI: Front Panel State>>%s" ("string"), w317) -> (resulting string=w316:string)  [unwired: 2 in, 1 out]
        n118 = call <vilib>:"Add State(s) to Queue__jki_lib_state_machine.vi"("State(s) in (\"\")"=w320, "State(s) at Back (\"\")"=w316) -> ("States Out"=w319:string)  [unwired: 13 in]
      }
      frame "CMD: Save Chart" {
        n119 = Unbundle By Name(w326) -> ("Indicator Refs.XY Graph"=w325:refnum<vi>)
        n120 = invoke class="XYGraph (strict)" method="Export Data to Excel"(reference=w325, error in=w324) -> (error out=w323:errorcluster)  [unwired: 1 in, 2 out]
      }
    }
  }
  "error out" <- w4
  "reference out" <- "reference in"
